vi "GetParam.vi"(8 "error in (no error)":errorcluster caption="entrée d'erreur (pas d'erreur)", 11 "Gaussian_Quantiles.lvclass":refnum<class "Gaussian_Quantiles.lvclass">) -> (0 "error out":errorcluster caption="sortie d'erreur", 2 "make_gaussian_quantiles":T1={"mean"=[-1.0], "cov "=1.0, "n_samples"=100, "n_features"=2, "n_classes"=3, "shuffle"=TRUE, "random_state"=-1, "Returns"="X"} {"random_state" min=-1; "n_classes" min=1; "n_features" min=1; "n_samples" min=1}, 3 "Gaussian_Quantiles.lvclass":refnum<class "Gaussian_Quantiles.lvclass">)   [LabVIEW 2020, in "Gaussian_Quantiles.lvclass"]
doc: "Get Parameters"
uses:
  Gaussian_Quantiles.lvclass
  Gaussian_Quantiles.lvclass/Gaussian_Quantiles.ctl
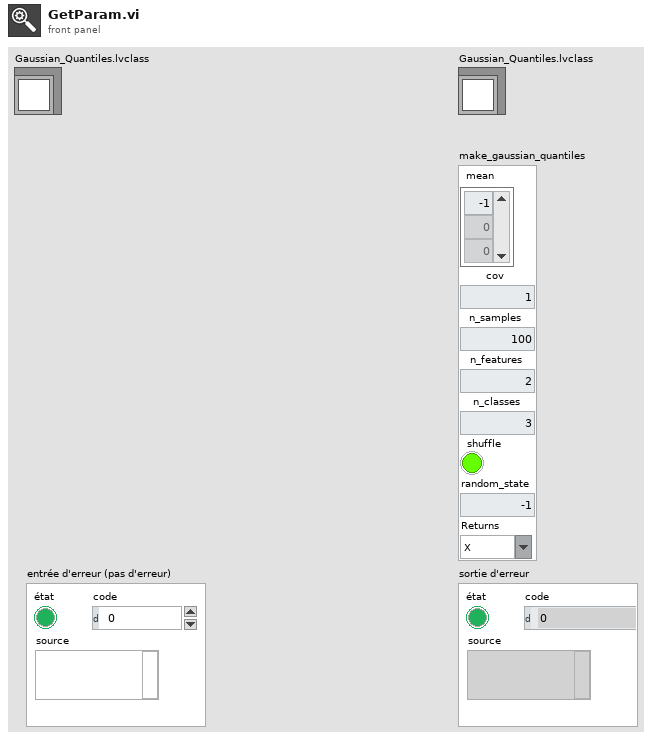
[diagram p1: front panel]
types:
  T1 = cluster{"mean":dbl[], "cov ":dbl, "n_samples":u32, "n_features":u32, "n_classes":u32, "shuffle":bool, "random_state":i32, "Returns":string}
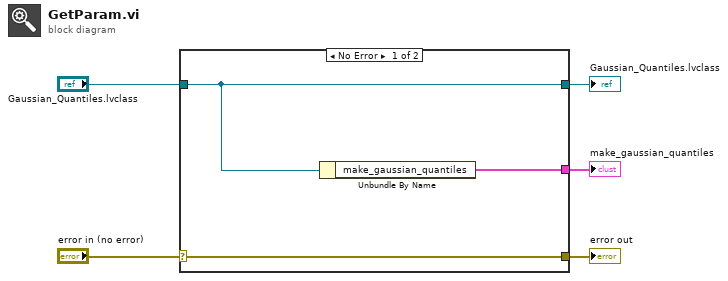
[diagram p0: block diagram]
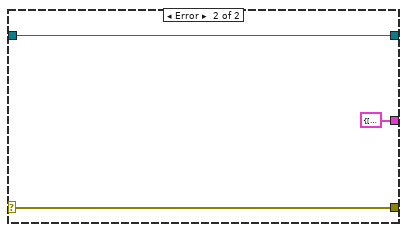
[diagram p2: hidden frame]
diagram:
  n1 = case shown="No Error" "error in (no error)" {
    selector: "error in (no error)" -> [w8 w10]
    tunnel: [w8 w10] -> w4
    tunnel: [w7 w11] -> w2
    tunnel: "Gaussian_Quantiles.lvclass" -> [w7 w11]
    tunnel: [w6 T1 {"mean"=[], "cov "=0.0, "n_samples"=0, "n_features"=0, "n_classes"=0, "shuffle"=FALSE, "random_state"=0, "Returns"=""} ("make_gaussian_quantiles")] -> w1
    frame No Error {
      n2 = Unbundle By Name(w7) -> ("make_gaussian_quantiles"=w6:T1)
    }
    frame Error {
    }
  }
  "error out" <- w4
  "Gaussian_Quantiles.lvclass" <- w2
  "make_gaussian_quantiles" <- w1
